vi "Test-Grabber-Direct Open-Close.vi"() -> ()   [LabVIEW 2014, in "Dev Grabber.lvlib"]
uses:
  Dev Grabber.lvlib
  Robot Actor Framework/Trace/Trace Controller Class/Config.ctl
  Dev Grabber Class/Dev Grabber Config.ctl
  <vilib>/Rock Robotics/WPI/Solenoid/WPI_SolenoidChannel.ctl
  Comp Robot/Comp Trace Controller/Comp Trace Controller Class/Comp Trace Controller.lvclass
  Comp Robot/Comp Pressure/Comp Pressure Class/Comp Pressure.lvclass
  Dev Grabber Class/Dev Grabber.lvclass
  <vilib>/Rock Robotics/WPI/DriverStation/WPI_DriverStationRobotMode2.ctl
  <vilib>/Rock Robotics/WPI/Solenoid/WPI_SolenoidValue.ctl
  Robot/Grabber/Grabber Messages/Spin Wheels Msg/Spin Wheels Msg.lvclass/Spin Wheels Msg.ctl
  <vilib>/ActorFramework/Message Enqueuer/Message Enqueuer.lvclass/Message Enqueuer.ctl
  <vilib>/ActorFramework/Message Enqueuer/Enqueue.vi
  <vilib>/Rock Robotics/WPI/Solenoid/WPI_SolenoidOpenDouble.vi
  <vilib>/Rock Robotics/WPI/Solenoid/WPI_SolenoidSetEnum.vi
  <vilib>/ActorFramework/Message Priority Queue/Priority Enqueue.vi
  Robot/Grabber/Grabber Messages/Spin Wheels Msg/Spin Wheels Msg.lvclass
  Robot/Grabber/Grabber Messages/Close Arms Msg/Close Arms Msg.lvclass
  Robot/Grabber/Grabber Messages/Open Arms Msg/Open Arms Msg.lvclass
  <vilib>/ActorFramework/Stop Msg/Stop Msg.lvclass
  <vilib>/ActorFramework/Actor/Actor.lvclass
  Robot Actor Framework/Trace/Trace Controller Class/Trace Controller.lvclass
panel:
  in  "Open Arms":bool=TRUE
  in  "Spin Direction":enum32{"Spin out", "Spin Off", "Spin In"}(radio)=enum."Spin Off"
  in  "Dev Grabber Config":T1={"PCM CAN ID"=3, "Forward Solenoid Channel"=enum."Solenoid 0", "Reverse Solenoid Channel"=enum."Solenoid 1", "Left Motor CAN ID"=13, "Right Motor CAN ID"=8, "Left Motor Invert"=FALSE, "Right Motor Invert"=TRUE}
  in  "Test Loop":u32=75
  out "Enable Tele":bool=TRUE caption="Enabled Teleop"
  in  "Stop Test Loop 1":bool=TRUE
  in  "Finish Test":bool=TRUE
  in  "Start Test":bool=TRUE
  in  "Trace Controller Config":T3={"Folder Pattern"="/media/sd%s1", "Starting Letter Position"=1, "Min Free Space (MB)"=50.0, "Max Folders to Check"=10, "Trace Level"=enum."Debug"} {"Min Free Space (MB)" format="%#_13g"}
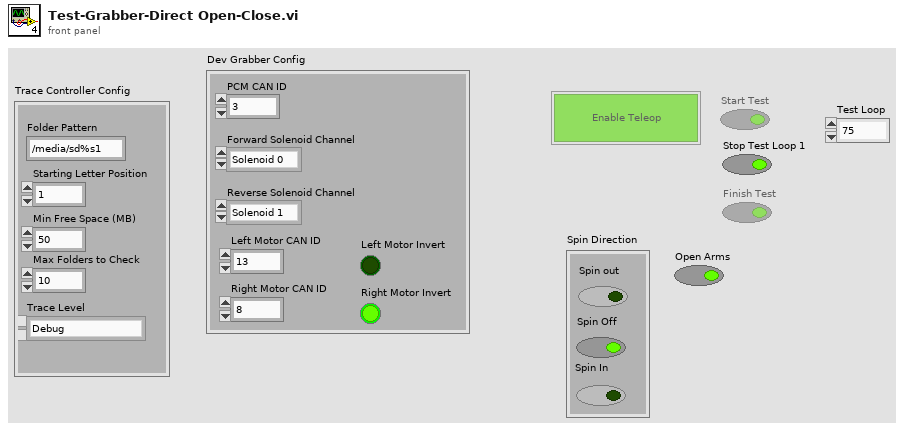
[diagram p1: front panel]
types:
  T1 = typedef "Dev Grabber.lvlib/Dev Grabber.lvclass/Dev Grabber Config.ctl" = cluster{"PCM CAN ID":u8, "Forward Solenoid Channel":T2, "Reverse Solenoid Channel":T2, "Left Motor CAN ID":u8, "Right Motor CAN ID":u8, "Left Motor Invert":bool, "Right Motor Invert":bool}
  T2 = typedef "WPI_SolenoidChannel.ctl" = enum8{"Solenoid 0", "Solenoid 1", "Solenoid 2", "Solenoid 3", "Solenoid 4", "Solenoid 5", "Solenoid 6", "Solenoid 7", "Invalid"}
  T3 = typedef "Robot Actor Framework.lvlib/Trace.lvlib/Trace Controller.lvclass/Config.ctl" = cluster{"Folder Pattern":string, "Starting Letter Position":i32, "Min Free Space (MB)":dbl, "Max Folders to Check":u32, "Trace Level":enum16{"Critical", "Error", "Warning", "Informational", "Debug"}}
  T4 = enum16{"Critical", "Error", "Warning", "Informational", "Debug"}
  T5 = enum8{"Enabled", "Disabled", "Disabled and Grayed Out"}
  T6 = typedef "WPI_DriverStationRobotMode2.ctl" = enum16{"Autonomous Disabled", "Autonomous Enabled", "Teleop Disabled", "Teleop Enabled", "Disconnected", "Finish", "Test Disabled", "Test Enabled", "Emergency Stopped"}
  T7 = typedef "WPI_SolenoidValue.ctl" = enum16{"Off", "On", "Forward", "Reverse"}
  T8 = typedef "WPI_SolenoidDevRef.ctl" = cluster{"DevStatus":errorcluster, "Pneumatics Control Module":u8, "Forward Solenoid Channel":T2, "Reverse Solenoid Channel":T2}
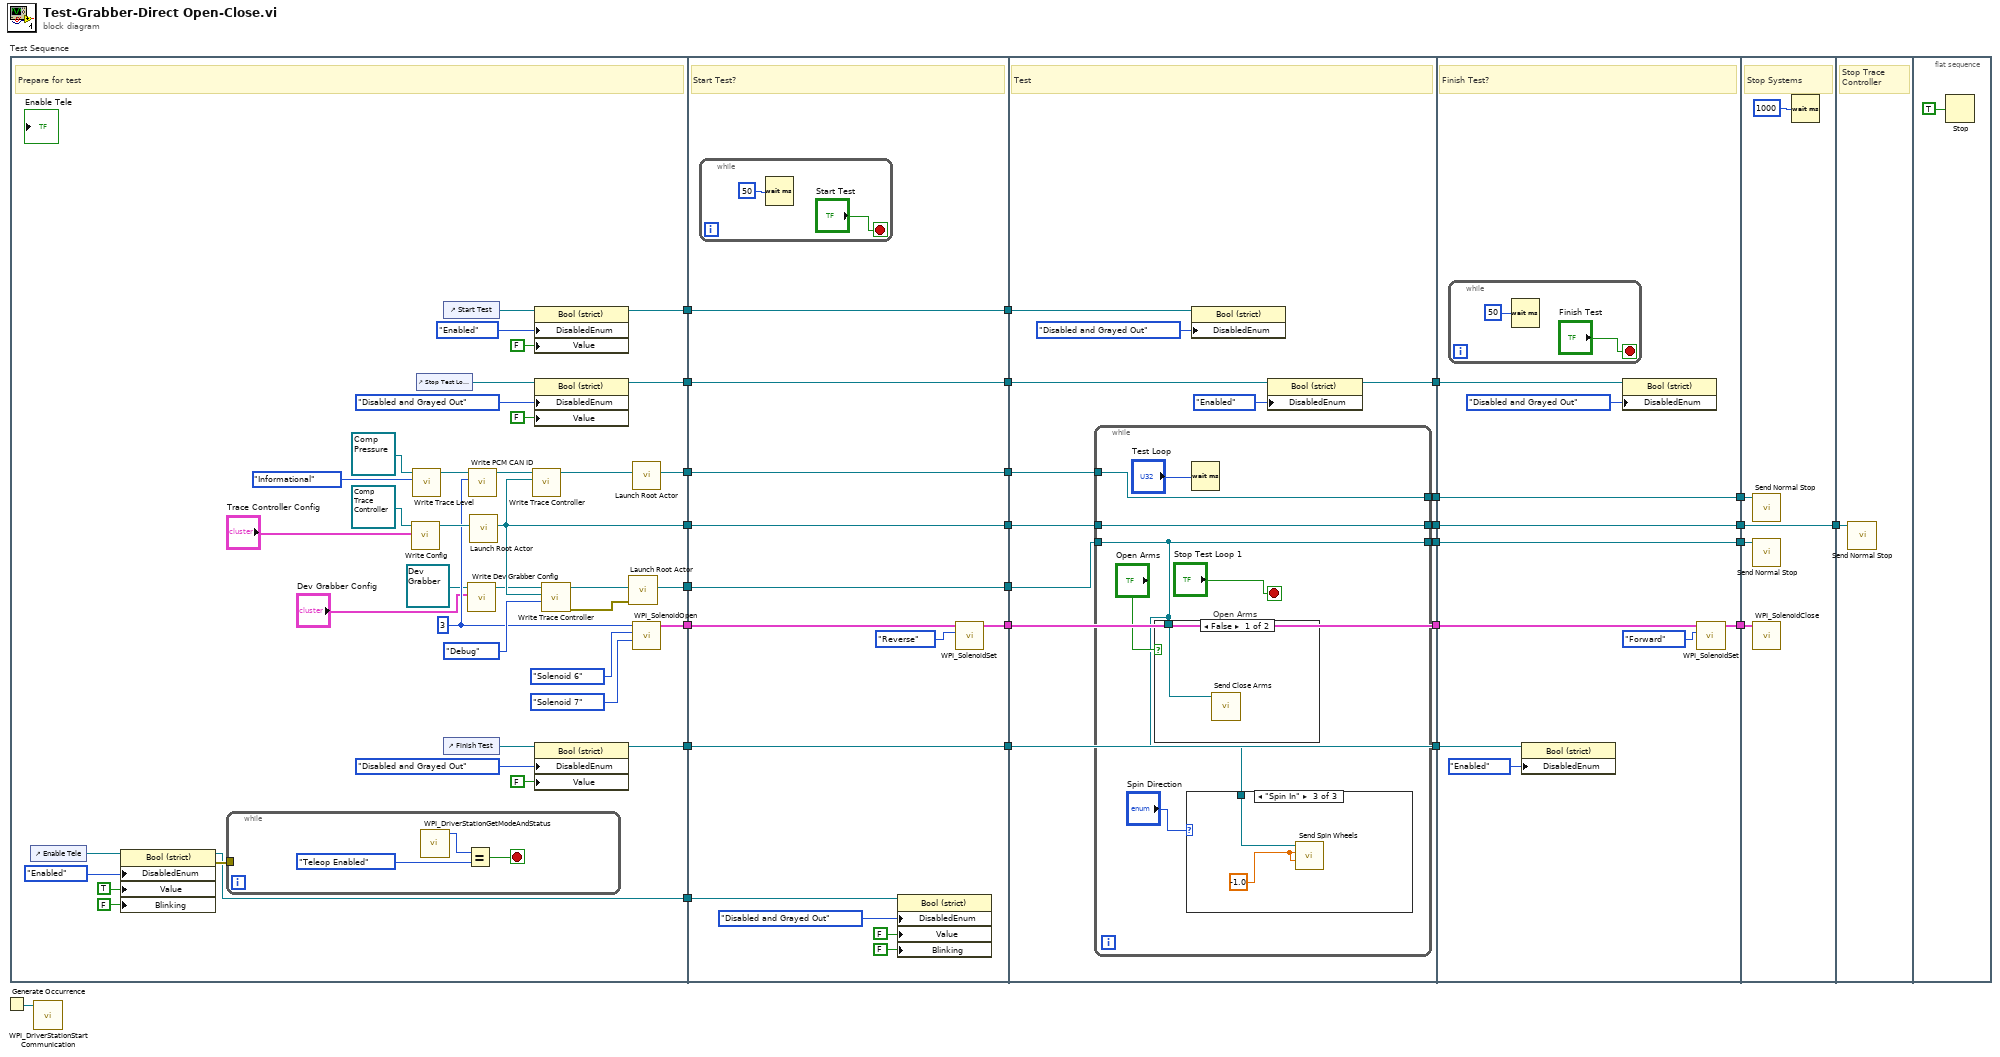
[diagram p0: block diagram]
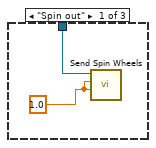
[diagram p2: hidden frame]
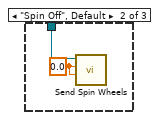
[diagram p3: hidden frame]
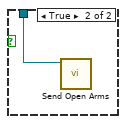
[diagram p4: hidden frame]
diagram:
  n1 = Generate Occurrence() -> (w27:refnum<k4>)
  n2 = flat-sequence "Test Sequence" {
    tunnel: [w54] -> w16
    tunnel: [w56] -> w15
    tunnel: [w55] -> w14
    tunnel: [w44] -> w13
    tunnel: [w43] -> w11
    tunnel: [w42] -> w6
    tunnel: [w36] -> w5
    tunnel: [w33] -> w4
    tunnel: [w82] -> w19
    tunnel: [w81] -> w18
    tunnel: [w80] -> w17
    tunnel: w16 -> [w82]
    tunnel: w15 -> [w81]
    tunnel: w14 -> [w80]
    tunnel: w13 -> [w79]
    tunnel: [w79] -> w12
    tunnel: w11 -> [w78]
    tunnel: [w78] -> w10
    tunnel: [w77] -> w7
    tunnel: w6 -> [w77]
    tunnel: w5 -> [w76]
    tunnel: w4 -> [w72]
    tunnel: [w71] -> w3
    tunnel: [w92] -> w22
    tunnel: [w94] -> w21
    tunnel: [w93] -> w20
    tunnel: w19 -> [w97]
    tunnel: w18 -> [w95]
    tunnel: w17 -> [w96]
    tunnel: w12 -> [w91]
    tunnel: w10 -> [w89]
    tunnel: [w87] -> w9
    tunnel: [w86] -> w8
    tunnel: w7 -> [w86]
    tunnel: w3 -> [w85]
    tunnel: [w85] -> w2
    tunnel: [w122] -> w25
    tunnel: [w121] -> w24
    tunnel: [w120] -> w23
    tunnel: w22 -> [w122]
    tunnel: w21 -> [w121]
    tunnel: w20 -> [w120]
    tunnel: w9 -> [w119]
    tunnel: w8 -> [w116]
    tunnel: w2 -> [w115]
    tunnel: [w114] -> w1
    tunnel: [w129] -> w26
    tunnel: w25 -> [w129]
    tunnel: w24 -> [w128]
    tunnel: w23 -> [w126]
    tunnel: w1 -> [w125]
    tunnel: w26 -> [w130]
    frame #0 {
      w34 = u8 3 ("PCM CAN ID")
      # "Prepare for test"
      n3 = control-ref of="Enable Tele"() -> (w41:refnum<vi>)
      n4 = property class="Bool (strict)"(reference=w41, "DisabledEnum"=T5."Enabled" ("Disabled"), "Value"=TRUE, "Blinking"=FALSE) -> (reference out=w36:refnum<vi>, error out=w38:errorcluster)  [unwired: 1 in]
      n5 = while {
        tunnel: w38 -> [_]
        stop <- w67 stop-if-true
        n6 = call <vilib>:"WPI_DriverStationGetModeAndStatus.vi"() -> ("Robot Mode"=w69:T6)  [unwired: 10 in, 1 out]
        n7 = Equal?(x=w69, y=WPI_DriverStationRobotMode2."Teleop Enabled") -> (x = y?=w67:bool)
      }
      n8 = call-dynamic "Write Config.vi"("Config"="Trace Controller Config", "Trace Controller in"=refnum<class "Comp Trace Controller.lvclass"> refnum ("Comp Trace Controller.lvlib:Comp Trace Controller.lvclass")) -> ("Trace Controller out"=w59:refnum<class "Comp Trace Controller.lvclass">)  [unwired: 8 in, 1 out]
      n9 = call-dynamic "Write Trace Level.vi"("Trace Level"=T4."Informational", "System Actor in"=refnum<class "Comp Pressure.lvclass"> refnum ("Comp Pressure.lvlib:Comp Pressure.lvclass")) -> ("System Actor out"=w64:refnum<class "Comp Pressure.lvclass">)  [unwired: 8 in, 1 out]
      n10 = control-ref of="Stop Test Loop 1"() -> (w48:refnum<vi>)
      n11 = control-ref of="Start Test"() -> (w53:refnum<vi>)
      n12 = control-ref of="Finish Test"() -> (w47:refnum<vi>)
      n13 = call-dynamic "Write Dev Grabber Config.vi"("Dev Grabber Config"="Dev Grabber Config", "Dev Grabber in"=refnum<class "Dev Grabber.lvclass"> refnum ("Dev Grabber.lvlib:Dev Grabber.lvclass")) -> ("Dev Grabber out"=w28:refnum<class "Dev Grabber.lvclass">)  [unwired: 8 in, 1 out]
      n14 = call-dynamic "Write PCM CAN ID.vi"("PCM CAN ID"=w34, "Comp Pressure in"=w64) -> ("Comp Pressure out"=w65:refnum<class "Comp Pressure.lvclass">)  [unwired: 8 in, 1 out]
      n15 = call <vilib>:"Launch Root Actor.vi"("Actor"=w59) -> ("Actor's Enqueuer"=w55:refnum<class "Message Enqueuer.lvclass">)  [unwired: 9 in, 1 out]
      n16 = call-dynamic "Write Trace Controller.vi"("Trace Controller"=w55, "System Actor in"=w65) -> ("System Actor out"=w66:refnum<class "Comp Pressure.lvclass">)  [unwired: 8 in, 1 out]
      n17 = property class="Bool (strict)"(reference=w53, "DisabledEnum"=T5."Enabled" ("Disabled"), "Value"=FALSE) -> (reference out=w44:refnum<vi>)  [unwired: 1 in, 1 out]
      n18 = property class="Bool (strict)"(reference=w48, "DisabledEnum"=T5."Disabled and Grayed Out" ("Disabled"), "Value"=FALSE) -> (reference out=w43:refnum<vi>)  [unwired: 1 in, 1 out]
      n19 = property class="Bool (strict)"(reference=w47, "DisabledEnum"=T5."Disabled and Grayed Out" ("Disabled"), "Value"=FALSE) -> (reference out=w42:refnum<vi>)  [unwired: 1 in, 1 out]
      n20 = call-dynamic "Write Trace Controller.vi"("Trace Level"=T4."Debug", "Trace Controller"=w55, "System Actor in"=w28) -> ("error out"=w61:errorcluster, "System Actor out"=w60:refnum<class "Dev Grabber.lvclass">)  [unwired: 7 in]
      n21 = call <vilib>:"Launch Root Actor.vi"("error in (no error)"=w61, "Actor"=w60) -> ("Actor's Enqueuer"=w54:refnum<class "Message Enqueuer.lvclass">)  [unwired: 8 in, 1 out]
      n22 = call <vilib>:"Launch Root Actor.vi"("Actor"=w66) -> ("Actor's Enqueuer"=w56:refnum<class "Message Enqueuer.lvclass">)  [unwired: 9 in, 1 out]
      n23 = call-poly <vilib>:"WPI_SolenoidOpen.vi"("Reverse Solenoid Channel"=WPI_SolenoidChannel."Solenoid 7", "Forward Solenoid Channel"=WPI_SolenoidChannel."Solenoid 6", "Pneumatics Control Module (0)"=w34) -> ("SolenoidDevRef"=w33:T8)  [unwired: 7 in, 1 out]
    }
    frame #1 {
      # "Start Test?"
      n24 = while {
        stop <- "Start Test" stop-if-true
        n25 = Wait (ms)(milliseconds to wait=u32 50) -> ()  [unwired: 1 out]
      }
      n26 = property class="Bool (strict)"(reference=w76, "DisabledEnum"=T5."Disabled and Grayed Out" ("Disabled"), "Value"=FALSE, "Blinking"=FALSE) -> ()  [unwired: 1 in, 2 out]
      n27 = call-poly <vilib>:"WPI_SolenoidSet.vi"("Value"=WPI_SolenoidValue."Reverse", "SolenoidDevRef"=w72) -> ("SolenoidDevRef"=w71:T8)  [unwired: 8 in, 1 out]
    }
    frame #2 {
      # "Test"
      n28 = while {
        tunnel: w96 -> [w103]
        tunnel: [w103] -> w92
        tunnel: w97 -> [w98]
        tunnel: [w98] -> w94
        tunnel: w95 -> [w102]
        tunnel: [w102] -> w93
        stop <- "Stop Test Loop 1" stop-if-true
        n29 = case "Open Arms" shown="False" "Open Arms" {
          tunnel: w98 -> [w111 w112]
          frame False {
            n30 = call "Send Close Arms.vi"("Message Enqueuer"=w111) -> ()  [unwired: 9 in, 2 out]
          }
          frame True {
            n31 = call "Send Open Arms.vi"("Message Enqueuer"=w112) -> ()  [unwired: 9 in, 2 out]
          }
        }
        n32 = case shown="\"Spin In\"" "Spin Direction" {
          tunnel: w98 -> [w106 w108 w110]
          frame "Spin out" {
            w105 = 1.0
            n33 = call "Send Spin Wheels.vi"("Right Wheel Power"=w105, "Left Wheel Power"=w105, "Message Enqueuer"=w106) -> ()  [unwired: 7 in, 2 out]
          }
          frame "Spin Off", Default {
            w107 = 0.0 ("Left Wheel Power")
            n34 = call "Send Spin Wheels.vi"("Right Wheel Power"=w107, "Left Wheel Power"=w107, "Message Enqueuer"=w108) -> ()  [unwired: 7 in, 2 out]
          }
          frame "Spin In" {
            w109 = -1.0
            n35 = call "Send Spin Wheels.vi"("Right Wheel Power"=w109, "Left Wheel Power"=w109, "Message Enqueuer"=w110) -> ()  [unwired: 7 in, 2 out]
          }
        }
        n36 = Wait (ms)(milliseconds to wait="Test Loop") -> ()  [unwired: 1 out]
      }
      n37 = property class="Bool (strict)"(reference=w91, "DisabledEnum"=T5."Disabled and Grayed Out" ("Disabled")) -> ()  [unwired: 1 in, 2 out]
      n38 = property class="Bool (strict)"(reference=w89, "DisabledEnum"=T5."Enabled" ("Disabled")) -> (reference out=w87:refnum<vi>)  [unwired: 1 in, 1 out]
    }
    frame #3 {
      # "Finish Test?"
      n39 = while {
        stop <- "Finish Test" stop-if-true
        n40 = Wait (ms)(milliseconds to wait=u32 50) -> ()  [unwired: 1 out]
      }
      n41 = property class="Bool (strict)"(reference=w116, "DisabledEnum"=T5."Enabled" ("Disabled")) -> ()  [unwired: 1 in, 2 out]
      n42 = property class="Bool (strict)"(reference=w119, "DisabledEnum"=T5."Disabled and Grayed Out" ("Disabled")) -> ()  [unwired: 1 in, 2 out]
      n43 = call-poly <vilib>:"WPI_SolenoidSet.vi"("Value"=WPI_SolenoidValue."Forward", "SolenoidDevRef"=w115) -> ("SolenoidDevRef"=w114:T8)  [unwired: 8 in, 1 out]
    }
    frame #4 {
      # "Stop Systems"
      n44 = call <vilib>:"Send Normal Stop.vi"("Message Enqueuer"=w126) -> ()  [unwired: 10 in, 1 out]
      n45 = call <vilib>:"Send Normal Stop.vi"("Message Enqueuer"=w128) -> ()  [unwired: 10 in, 1 out]
      n46 = call <vilib>:"WPI_SolenoidClose.vi"("SolenoidDevRef"=w125) -> ()  [unwired: 10 in, 1 out]
      n47 = Wait (ms)(milliseconds to wait=u32 1000) -> ()  [unwired: 1 out]
    }
    frame #5 {
      # "Stop Trace Controller"
      n48 = call <vilib>:"Send Normal Stop.vi"("Message Enqueuer"=w130) -> ()  [unwired: 10 in, 1 out]
    }
    frame #6 {
      n49 = Stop(stop? (T)=TRUE) -> ()
    }
  }
  n50 = call <vilib>:"WPI_DriverStationStart Communication.vi"("occurrence"=w27) -> ()  [unwired: 1 in, 10 out]
